vi "Лабораторная №1 Задание 3_9.vi"() -> ()   [LabVIEW 2017]
panel:
  out "Meter":dbl(knob) scale=-1.0..10.0
  in  "Knob":dbl(knob) scale=0.0..10.0
  in  "Boolean":bool
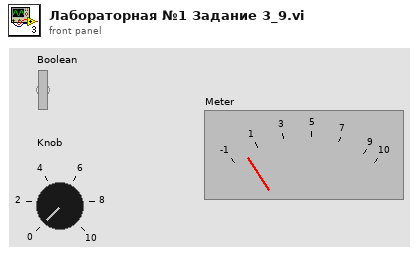
[diagram p1: front panel]
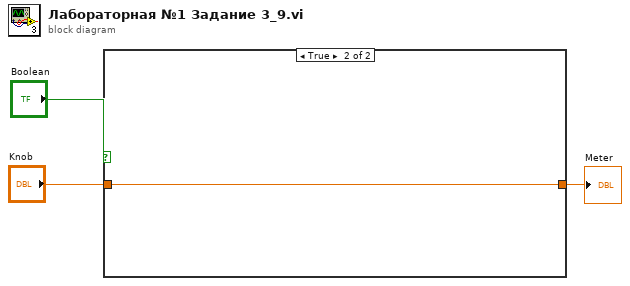
[diagram p0: block diagram]
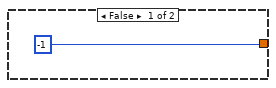
[diagram p2: hidden frame]
diagram:
  n1 = case shown="True" "Boolean" {
    tunnel: "Knob" -> [_ w5]
    tunnel: [-1 w5] -> w1
    frame False {
    }
    frame True {
    }
  }
  "Meter" <- w1
